vi "Image Generator.vi"(6 "Hide Labels":bool, 7 "Lithography Data":T2(array[cluster]), 8 "error in (no error)":errorcluster, 9 "Resolution":i32=444, 11 "Image Reference In":T3) -> (0 "error out":errorcluster, 3 "Image Reference Out":T3)   [LabVIEW 2019]
doc: "This VI generates a rendered image given the lithography data."
uses:
  <vilib>/vision/Image Controls.llb/IMAQ Image.ctl
  <userlib>/LevyLab/Relay Box/Typedefs/Resistor--enum.ctl
  <userlib>/LevyLab/Relay Box/Relay-Box.lvclass
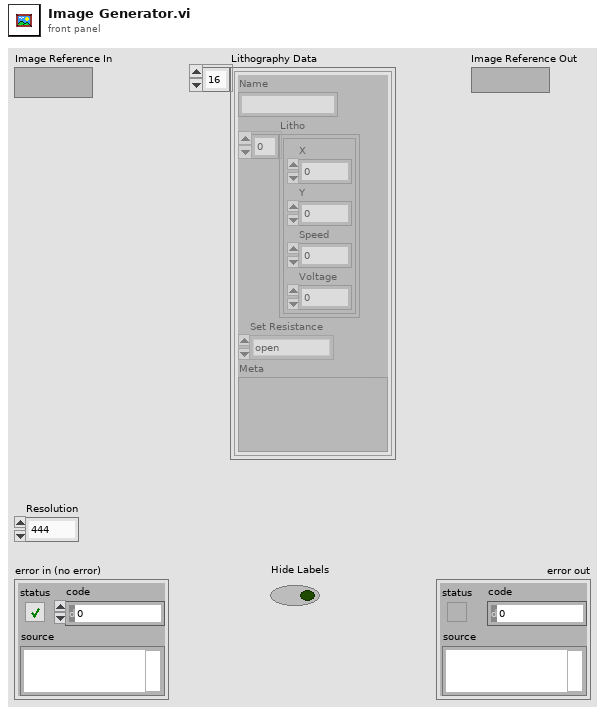
[diagram p1: front panel]
types:
  T1 = typedef "Relay-Box.lvclass/Resistor--enum.ctl" = enum16{"open", "discharge tip", "0 ohms", "100k ohm", "10M ohm", "1G ohm"}
  T2 = cluster{"Name":string, "Litho":cluster{"X":dbl, "Y":dbl, "Speed":dbl, "Voltage":dbl}[], "Set Resistance":T1, "Meta":variant}[]
  T3 = typedef "IMAQ Image.ctl" = refnum<image>
  T4 = cluster{"Desired Font (Application)":enum16{"User-specified Font", "Application Font", "System Font", "Dialog Font"}, "[User-specified Font]":cluster{"Font Name":string, "Size":i16, "Strikeout?":bool, "Italic?":bool, "Underline?":bool, "Outline?":bool, "Shadow?":bool, "Bold?":bool, "Rotation Angle":dbl}, "Horizontal Alignment":i16, "Vertical Alignment":i16}
  T5 = cluster{"Left":i32, "Top":i32, "Right":i32, "Bottom":i32}
  T6 = cluster{"X":dbl, "Y":dbl, "Speed":dbl, "Voltage":dbl}[]
  T7 = cluster{"X":dbl, "Y":dbl, "Speed":dbl, "Voltage":dbl}
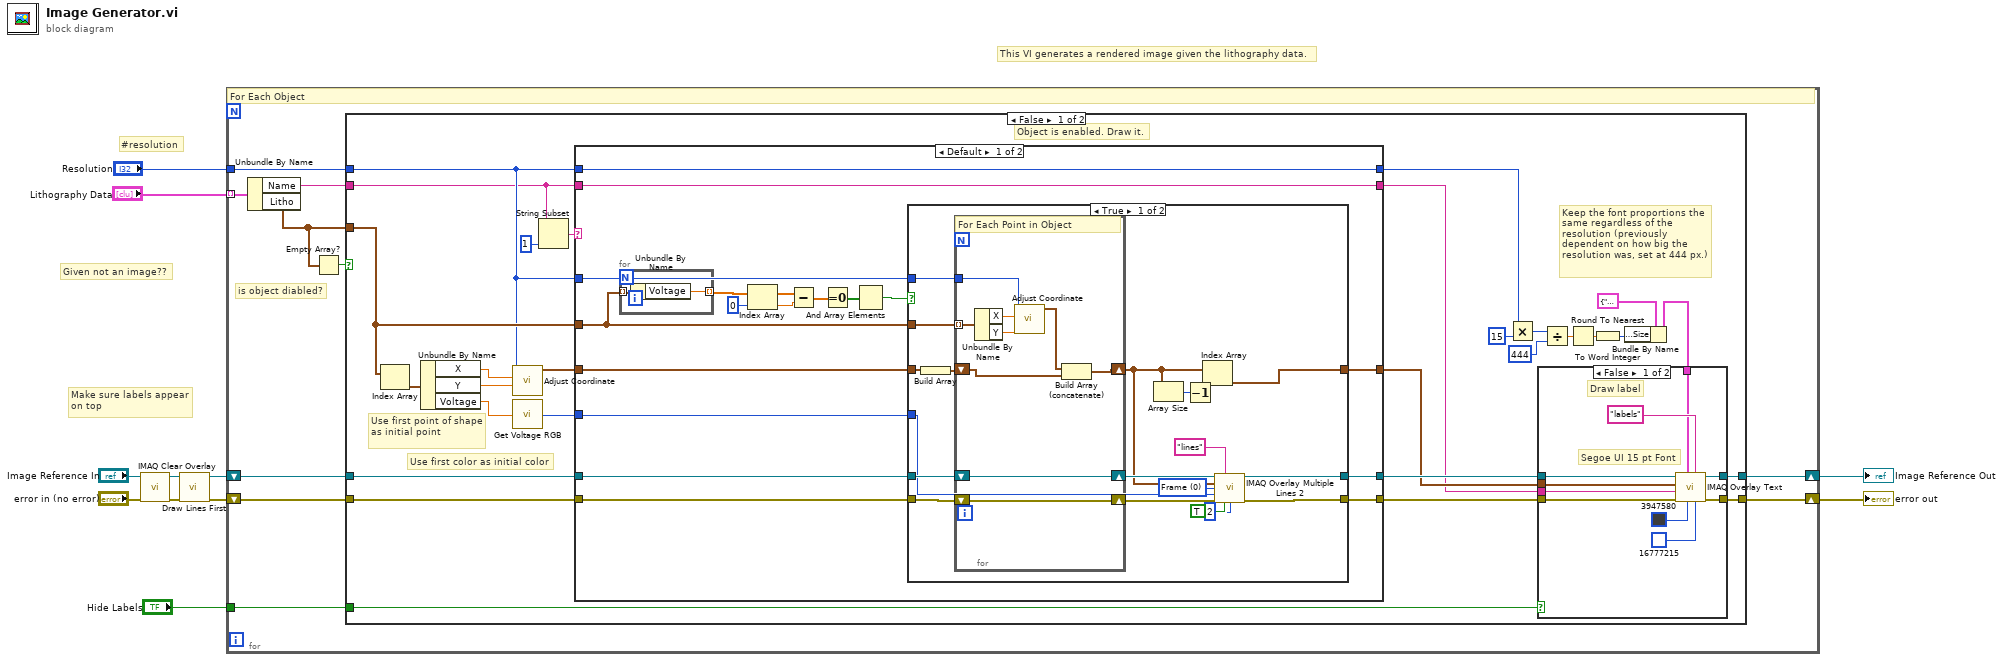
[diagram p0: block diagram]
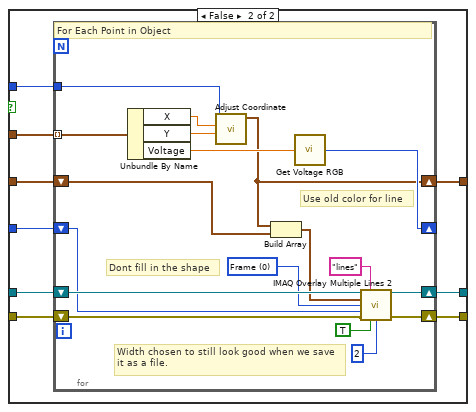
[diagram p3: hidden frame]
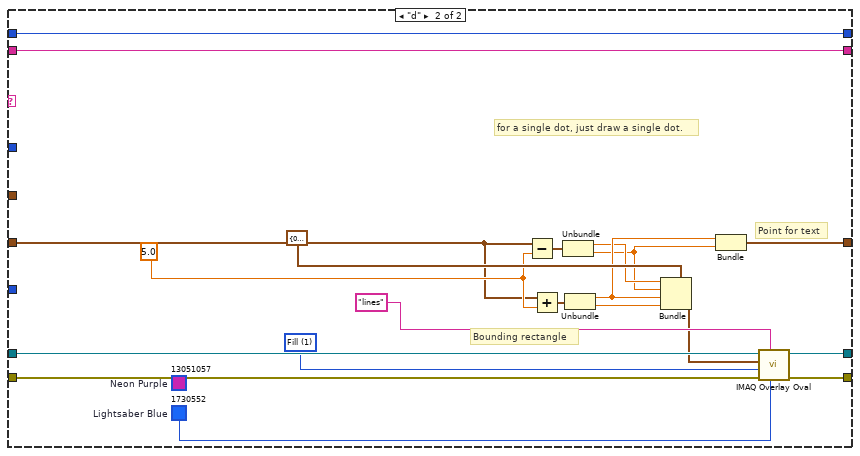
[diagram p4: hidden frame]
diagram:
  # "#resolution"
  # "Given not an image??"
  # "This VI generates a rendered image given the lithography data."
  # "Make sure labels appear\non top"
  n1 = call "IMAQ Clear Overlay"("error in (no error)"="error in (no error)", "Image"="Image Reference In") -> ("error out"=w4:errorcluster, "Image Out"=w5:T3)  [unwired: 8 in]
  n2 = call "Draw Lines First.vi"("error in (no error)"=w4, "Refnum in"=w5) -> ("error out"=w9:errorcluster, "Refnum out"=w10:T3)  [unwired: 8 in]
  n3 = for {
    tunnel: "Lithography Data" -> [w19] mode=indexing
    shift-right: [w20] -> w11
    shift-left: w9 -> [w21]
    tunnel: "Resolution" -> [w17]
    tunnel: "Hide Labels" -> [w13]
    shift-right: [w12] -> w1
    shift-left: w10 -> [w18]
    # "is object diabled?"
    # "For Each Object"
    n4 = Unbundle By Name(w19) -> ("Name"=w16:string, "Litho"=w14:T6)
    n5 = Empty Array?(array=w14) -> (empty?=w15:bool)
    n6 = case shown="False" w15 {
      tunnel: w21 -> [w50 w157]
      tunnel: [w48 w157] -> w20
      tunnel: [w46 w158] -> w12
      tunnel: w14 -> [w45 _]
      tunnel: w18 -> [w37 w158]
      tunnel: w17 -> [w28 _]
      tunnel: w16 -> [w25 _]
      tunnel: w13 -> [w22 _]
      frame False {
        # "Object is enabled. Draw it."
        # "Keep the font proportions the same regardless of the resolution (previously dependent on how big the resolution was, set at 444 px.)"
        # "Use first color as initial color"
        # "Use first point of shape as initial point"
        n7 = Index Array(array=w45) -> (element=w44:T7)  [unwired: 1 in]
        n8 = Unbundle By Name(w44) -> ("X"=w42:dbl, "Y"=w41:dbl, "Voltage"=w43:dbl)
        n9 = call "Adjust Coordinate.vi"("Y"=w41, "X"=w42, "Resolution"=w28) -> ("Adjusted Coordinate"=w39:cluster{dbl, dbl})  [unwired: 7 in, 1 out]
        n10 = call "Get Voltage RGB.vi"("Voltage"=w43) -> ("RGB Value"=w40:u32)  [unwired: 3 in, 1 out]
        n11 = String Subset(string=w25, length (rest)=1 ("length (rest)")) -> (substring=w23:string)  [unwired: 1 in]
        n12 = case shown="Default" w23 {
          tunnel: w50 -> [w79 w140]
          tunnel: [w78 w154] -> w49
          tunnel: [w77 w153] -> w47
          tunnel: w45 -> [w69 _]
          tunnel: w40 -> [w76 _]
          tunnel: w39 -> [w75 w138]
          tunnel: [w74 w137] -> w38
          tunnel: w37 -> [w73 w152]
          tunnel: w28 -> [w72 _]
          tunnel: w25 -> [w71 w155]
          tunnel: w28 -> [w70 w156]
          tunnel: [w71 w155] -> w27
          tunnel: [w70 w156] -> w26
          frame Default {
            n13 = for {
              tunnel: w69 -> [w136] mode=indexing
              tunnel: [w135] -> w67 mode=indexing
              n14 = Unbundle By Name(w136) -> ("Voltage"=w135:dbl)
            }
            n15 = Index Array(array=w67, index=0) -> (element=w66:dbl)
            n16 = Subtract(x=w67, y=w66) -> (x-y=w65:dbl[])
            n17 = Equal To 0?(x=w65) -> (x = 0?=w64:bool[])
            n18 = And Array Elements(Boolean array=w64) -> (logical AND=w63:bool)
            n19 = case shown="True" w63 {
              tunnel: w79 -> [w98 w116]
              tunnel: [w93 w115] -> w78
              tunnel: [w91 w114] -> w77
              tunnel: w76 -> [w88 w113]
              tunnel: w75 -> [w81 w112]
              tunnel: [w83 w108] -> w74
              tunnel: w73 -> [w97 w111]
              tunnel: w72 -> [w96 w110]
              tunnel: w69 -> [w95 w109]
              frame True {
                w89 = u32 0 items=["Frame", "Fill"] ("Drawing Mode (Frame)")
                n20 = Build Array(w81) -> (w80:cluster{dbl, dbl}[])
                n21 = for {
                  tunnel: w95 -> [w107] mode=indexing
                  shift-right: [w102] -> w92
                  shift-left: w97 -> [w102]
                  shift-right: [w101] -> w94
                  shift-left: w98 -> [w101]
                  shift-right: [w99] -> w82
                  shift-left: w80 -> [w103]
                  tunnel: w96 -> [w104]
                  # "For Each Point in Object"
                  n22 = Unbundle By Name(w107) -> ("X"=w106:dbl, "Y"=w105:dbl)
                  n23 = call "Adjust Coordinate.vi"("Y"=w105, "X"=w106, "Resolution"=w104) -> ("Adjusted Coordinate"=w100:cluster{dbl, dbl})  [unwired: 7 in, 1 out]
                  n24 = Build Array (concatenate)(w100, w103) -> (w99:cluster{dbl, dbl}[])
                }
                n25 = Array Size(array=w82) -> (size(s)=w85:i32)
                n26 = Decrement(x=w85) -> (x-1=w84:i32)
                n27 = Index Array(array=w82, index=w84) -> (element=w83:cluster{dbl, dbl})
                n28 = call "IMAQ Overlay Multiple Lines 2"("Image"=w92, "Group"="lines", "Line End Points"=w82, "Drawing Mode (Frame)"=w89, "Color"=w88, "error in (no error)"=w94, "Maintain Width?"=TRUE, "Width"=u32 2) -> ("Image Out"=w91:T3, "error out"=w93:errorcluster)  [unwired: 6 in]
              }
              frame False {
                n29 = for {
                  tunnel: w109 -> [w132] mode=indexing
                  shift-right: [w134] -> w114
                  shift-left: w111 -> [w128]
                  shift-right: [w133] -> w115
                  shift-left: w116 -> [w123]
                  shift-right: [w127] -> _
                  shift-left: w113 -> [w119]
                  shift-right: [w121] -> w108
                  shift-left: w112 -> [w122]
                  tunnel: w110 -> [w126]
                  w117 = u32 0 items=["Frame", "Fill"] ("Drawing Mode (Frame)")
                  # "Dont fill in the shape"
                  # "Width chosen to still look good when we save it as a file."
                  # "Use old color for line"
                  # "For Each Point in Object"
                  n30 = Unbundle By Name(w132) -> ("X"=w130:dbl, "Y"=w129:dbl, "Voltage"=w131:dbl)
                  n31 = call "Adjust Coordinate.vi"("Y"=w129, "X"=w130, "Resolution"=w126) -> ("Adjusted Coordinate"=w121:cluster{dbl, dbl})  [unwired: 7 in, 1 out]
                  n32 = Build Array(w121, w122) -> (w120:cluster{dbl, dbl}[])
                  n33 = call "Get Voltage RGB.vi"("Voltage"=w131) -> ("RGB Value"=w127:u32)  [unwired: 3 in, 1 out]
                  n34 = call "IMAQ Overlay Multiple Lines 2"("Image"=w128, "Group"="lines", "Line End Points"=w120, "Drawing Mode (Frame)"=w117, "Color"=w119, "error in (no error)"=w123, "Maintain Width?"=TRUE, "Width"=u32 2) -> ("Image Out"=w134:T3, "error out"=w133:errorcluster)  [unwired: 6 in]
                }
              }
            }
          }
          frame "d" {
            w139 = u32 1730552  # Lightsaber Blue
            (unwired) u32 13051057  # Neon Purple
            w146 = u32 1 items=["Frame", "Fill"] ("Drawing Mode (Frame)")
            w144 = 5.0
            # "Point for text"
            # "Bounding rectangle"
            # "for a single dot, just draw a single dot."
            n35 = Subtract(x=w138, y=w144) -> (x-y=w149:cluster{dbl, dbl})
            n36 = Add(x=w138, y=w144) -> (x+y=w147:cluster{dbl, dbl})
            n37 = Unbundle(w149) -> (w142:dbl, w141:dbl)
            n38 = Unbundle(w147) -> (w143:dbl, w145:dbl)
            n39 = Bundle(cluster=T5 {"Left"=0, "Top"=0, "Right"=0, "Bottom"=0} ("Bounding Rectangle"), "Left"=w142, "Top"=w141, "Right"=w143, "Bottom"=w145) -> (w148:T5)
            n40 = Bundle(w143, w141) -> (w137:cluster{dbl, dbl})  [unwired: 1 in]
            n41 = call "IMAQ Overlay Oval"("Color"=w139, "Group"="lines", "error in (no error)"=w140, "Drawing Mode (Frame)"=w146, "Bounding Rectangle"=w148, "Image"=w152) -> ("error out"=w154:errorcluster, "Image Out"=w153:T3)  [unwired: 4 in]
          }
        }
        n42 = Multiply(x=w26, y=15) -> (x*y=w33:i32)
        n43 = Divide(x=w33, y=444) -> (x/y=w31:dbl)
        n44 = Round To Nearest(number=w31) -> (nearest integer value=w30:dbl)
        n45 = To Word Integer(number=w30) -> (16bit integer=w29:i16)
        n46 = Bundle By Name(cluster=T4 {"Desired Font (Application)"=enum."User-specified Font", "[User-specified Font]"={"Font Name"="Segoe UI", "Size"=35, "Strikeout?"=FALSE, "Italic?"=FALSE, "Underline?"=FALSE, "Outline?"=FALSE, "Shadow?"=FALSE, "Bold?"=FALSE, "Rotation Angle"=0.0}, "Horizontal Alignment"=0, "Vertical Alignment"=0} ("Font, Size & Style"), "[User-specified Font].Size"=w29) -> (w35:T4)
        n47 = case shown="False" w22 {
          tunnel: w49 -> [w60 w62]
          tunnel: [w59 w62] -> w48
          tunnel: w47 -> [w58 w61]
          tunnel: [w57 w61] -> w46
          tunnel: w38 -> [w51 _]
          tunnel: w35 -> [w53 _]
          tunnel: w27 -> [w52 _]
          frame False {
            # "Segoe UI 15 pt Font"
            # "Draw label"
            n48 = call "IMAQ Overlay Text"("BG Color (Transparent)"=u32 16777215, "Group"="labels", "Text Color (black)"=u32 3947580, "Font, Size & Style"=w53, "error in (no error)"=w60, "String"=w52, "Origin"=w51, "Image"=w58) -> ("error out"=w59:errorcluster, "Image Out"=w57:T3)  [unwired: 2 in]
          }
          frame True {
          }
        }
      }
      frame True {
        # "Object is disabled. Dont draw."
      }
    }
  }
  "Image Reference Out" <- w1
  "error out" <- w11
